vi "Find All Actors In Project.vi"(8 "error in (no error)":errorcluster, 9 "Include Dependencies?":bool, 11 "Message Maker in":refnum<class "Message Maker.lvclass">) -> (0 "error out":errorcluster, 2 "Actor Classes":refnum<vi>[](array[refnum]), 3 "Message Maker out":refnum<class "Message Maker.lvclass">)   [LabVIEW 2023, in "Message Maker.lvclass"]
doc: "Finds all actors in the project\n\nAuthor: Derek Trepanier\nCopyright: MGI 2015"
uses:
  Message Maker.lvclass
  Message Maker.lvclass/Message Maker.ctl
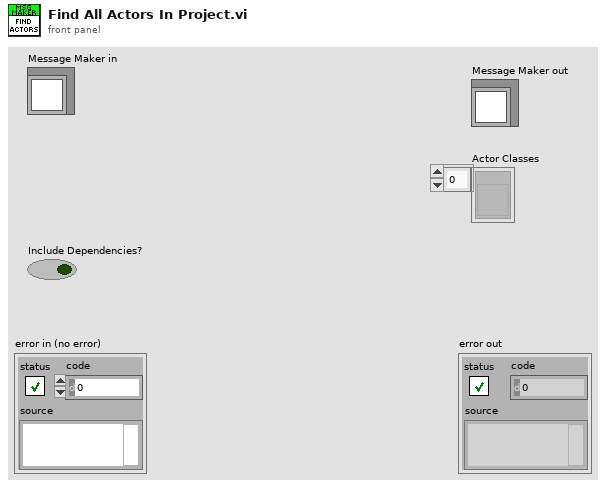
[diagram p1: front panel]
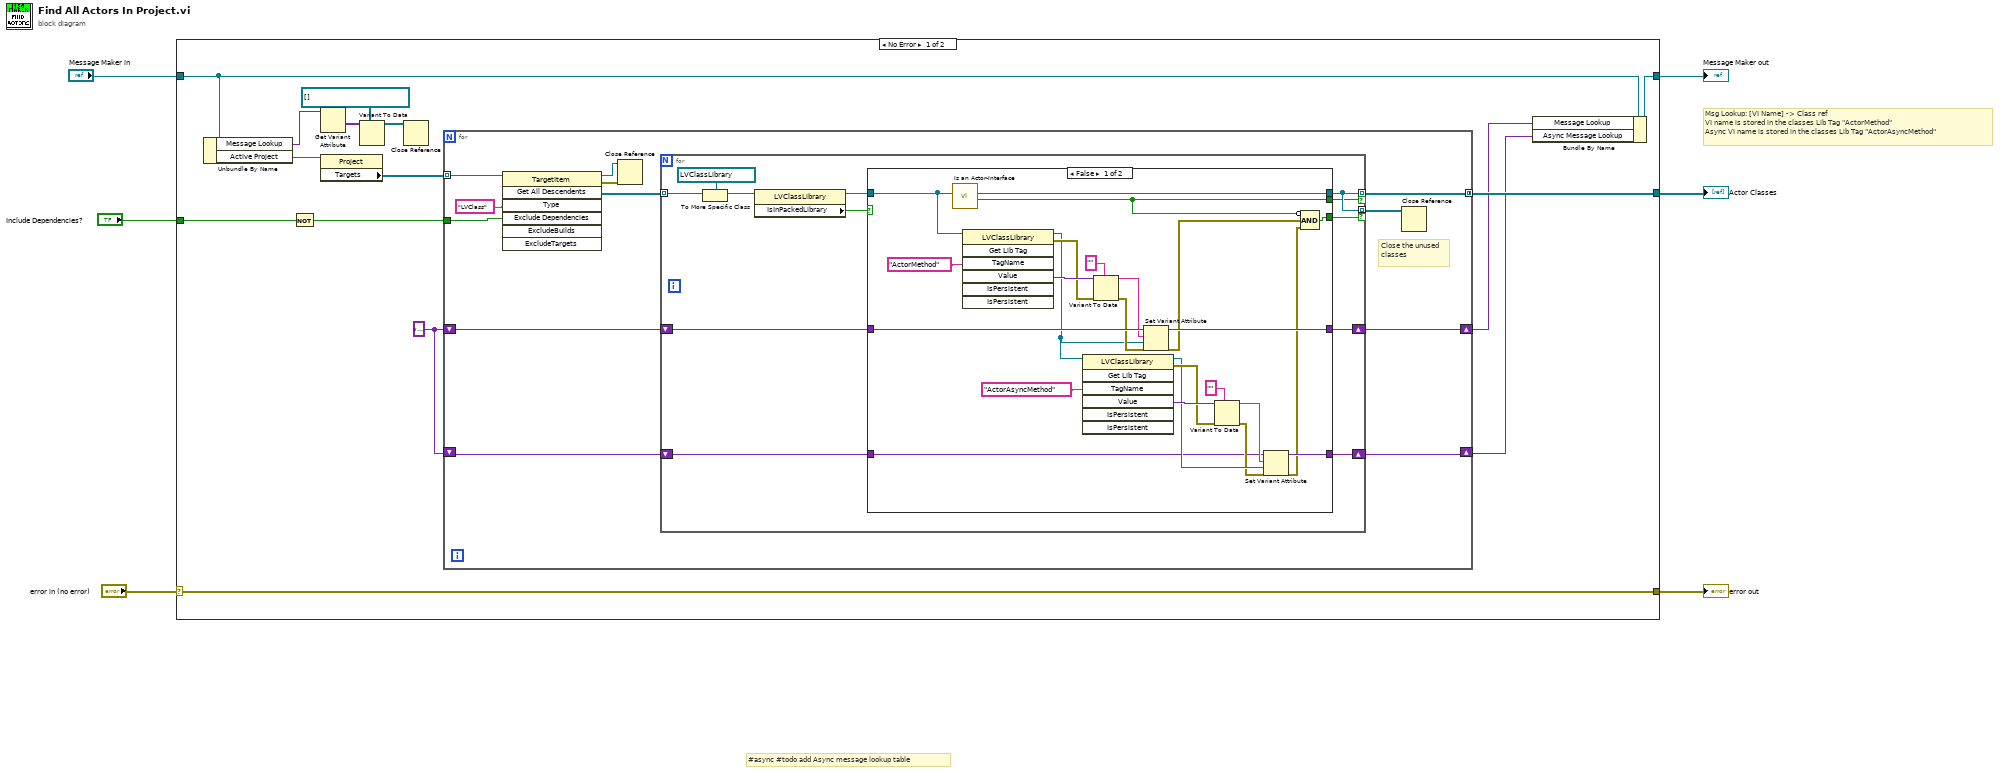
[diagram p0: block diagram]
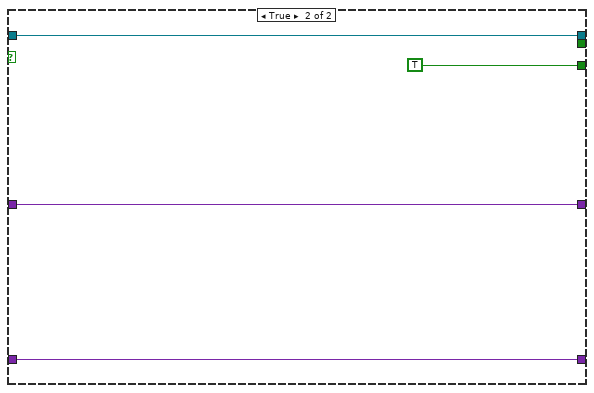
[diagram p2: hidden frame]
diagram:
  # "#async #todo add Async message lookup table"
  # "Msg Lookup: [VI Name] -> Class ref\nVI name is stored in the classes Lib Tag \"ActorMethod\"\nAsync VI name is stored in the classes Lib Tag \"ActorAsyncMethod\""
  n1 = case shown="No Error" "error in (no error)" {
    selector: "error in (no error)" -> [w21 w75]
    tunnel: [w21 w75] -> w5
    tunnel: "Include Dependencies?" -> [w19 _]
    tunnel: [w18 _] -> w3
    tunnel: "Message Maker in" -> [w17 w74]
    tunnel: [w15 w74] -> w1
    frame No Error {
      w8 = variant ("Value")
      n2 = Unbundle By Name(w17) -> ("Message Lookup"=w9:variant, "Active Project"=w16:refnum<vi>)
      n3 = Not(x=w19) -> (.not. x?=w10:bool)
      n4 = Get Variant Attribute(Variant=w9) -> (values=w13:variant[])  [unwired: 3 in, 3 out]
      n5 = property class="Project"(reference=w16) -> ("Targets"=w20:refnum<vi>[])  [unwired: 1 in, 2 out]
      n6 = Variant To Data(type=refnum<vi>[] [], Variant=w13) -> (data=w11:refnum<vi>[])  [unwired: 1 in, 1 out]
      n7 = Close Reference(reference=w11) -> ()  [unwired: 1 in, 1 out]
      n8 = for {
        tunnel: w20 -> [w33] mode=indexing
        shift-right: [w27] -> w14
        shift-left: w8 -> [w28]
        tunnel: w10 -> [w31]
        tunnel: [w29] -> w18 mode=concatenating
        shift-right: [w22] -> w7
        shift-left: w8 -> [w23]
        # "Close the unused classes"
        n9 = invoke class="TargetItem" method="Get All Descendents"(reference=w33, "Type"="LVClass", "Exclude Dependencies"=w31) -> (reference out=w24:refnum<vi>, error out=w25:errorcluster, "All Descendents"=w30:refnum<vi>[])  [unwired: 4 in, 4 out]
        n10 = Close Reference(reference=w24, error in (no error)=w25) -> ()  [unwired: 1 out]
        n11 = for {
          tunnel: w30 -> [w45] mode=indexing
          tunnel: [w39] -> w29 mode=indexing if=w38
          shift-right: [w42] -> w27
          shift-left: w28 -> [w43]
          tunnel: [w39] -> w26 mode=indexing if=w41
          shift-right: [w34] -> w22
          shift-left: w23 -> [w35]
          n12 = To More Specific Class(target class=refnum<vi> refnum ("reference out"), reference=w45) -> (specific class reference=w40:refnum<vi>)  [unwired: 1 in, 1 out]
          n13 = property class="LVClassLibrary"(reference=w40) -> (reference out=w37:refnum<vi>, "IsInPackedLibrary"=w36:bool)  [unwired: 1 in, 1 out]
          n14 = case shown="False" w36 {
            tunnel: w43 -> [w67 w71]
            tunnel: [w66 w71] -> w42
            tunnel: [w61 TRUE] -> w41
            tunnel: [w59 w73] -> w39
            tunnel: [w58 _] -> w38
            tunnel: w37 -> [w57 w73]
            tunnel: w35 -> [w49 w70]
            tunnel: [w48 w70] -> w34
            frame False {
              n15 = call "Is an Actor-Interface.vi"("Class in"=w57) -> ("Is Actor/Interface?"=w58:bool, "Class out"=w59:refnum<vi>)  [unwired: 7 in, 2 out]
              n16 = invoke class="LVClassLibrary" method="Get Lib Tag"(reference=w57, "TagName"="ActorMethod" ("Tag Name")) -> (reference out=w47:refnum<vi>, error out=w64:errorcluster, "Value"=w68:variant)  [unwired: 5 in, 4 out]
              n17 = invoke class="LVClassLibrary" method="Get Lib Tag"(reference=w47, "TagName"="ActorAsyncMethod" ("Tag Name")) -> (reference out=w51:refnum<vi>, error out=w53:errorcluster, "Value"=w55:variant)  [unwired: 5 in, 4 out]
              n18 = Variant To Data(error in=w64, type="" ("Tag Name"), Variant=w68) -> (data=w65:string, error out=w62:errorcluster)
              n19 = Set Variant Attribute(Variant=w67, name=w65, value=w47, error in=w62) -> (Variant out=w66:variant, error out=w60:errorcluster)  [unwired: 1 out]
              n20 = Variant To Data(error in=w53, type="" ("Tag Name"), Variant=w55) -> (data=w54:string, error out=w50:errorcluster)
              n21 = Set Variant Attribute(Variant=w49, name=w54, value=w51, error in=w50) -> (Variant out=w48:variant, error out=w46:errorcluster)  [unwired: 1 out]
              n22 = Compound Arithmetic op=AND(invert w58, w60, w46) -> (w61:bool)
            }
            frame True {
            }
          }
        }
        n23 = Close Reference(reference=w26) -> ()  [unwired: 1 in, 1 out]
      }
      n24 = Bundle By Name(cluster=w17, "Message Lookup"=w14, "Async Message Lookup"=w7) -> (w15:refnum<class "Message Maker.lvclass">)
    }
    frame Error {
    }
  }
  "error out" <- w5
  "Actor Classes" <- w3
  "Message Maker out" <- w1
